vi "Read File+ [I16].vi"(6 "2D number of columns/1D count":i32 caption="2D-Spaltenanzahl/1D-Anzahl", 7 "2D number of rows":i32 caption="2D-Zeilenanzahl", 8 "error in (no error)":errorcluster caption="Fehler (Eingang, kein Fehler)", 9 "pos offset (bytes:0)":i32 caption="Pos.-Offset (Bytes:0)", 10 "pos mode (rel. to current:2)":enum16{"start", "end", "current"}(ring)=enum."current" caption="Pos.-Modus (relativ zur aktuellen Pos.:2)", 11 "refnum":refnum<file> caption="RefNum") -> (0 "error out":errorcluster caption="Fehler (Ausgang)", 1 "mark after read (bytes)":i32 caption="Dateimarke nach Lesevorgang (Byte)", 2 "1D data":i16[](array[numeric]) caption="1D Daten", 3 "2D data":i16[][](array[numeric]) caption="2D Daten", 4 "EOF?":bool caption="Dateiende?", 5 "dup refnum":refnum<file> caption="RefNum (Kopie)")   [LabVIEW 2009]
doc: "Liest ein 2D- oder 1D-Array von vorzeichenbehafteten Word-Integerzahlen (I16) an der angegebenen Position einer Byte-Stream-Datei aus; der voreingestellte Ort ist die aktuelle Markierung. Das VI überprüft eingehende und interne Fehler und liest nicht, wenn ein Eingangsfehler auftritt.\n\n'RefNum' ist die Referenz zur geöffneten Datei.\n\n'Pos.-Modus' legt fest, an welcher Stelle, relativ zu 'Pos.-Offset', zu schreiben begonnen wird:\n\n 0: am Anfang der Datei plus Pos.-Offest.\n\n 1: am Ende der Datei plus Pos.-Offest. \n\n 2: An der aktuellen Markierung plus Pos.-Offset. Dies ist die Standardeinstellung\n\nPos.-Offset legt in Byte fest, wie weit entfernt von Pos.-Modus begonnen wird. Die Voreinstellung ist 0. Byte-Einheiten sind flexibler als Integer(2 Byte)-Einheiten, Wenn eine Datei zum Beispiel einen Kopf, geschrieben mit Datei Schreiben+ (String) enthält, gefolgt von Array mit Zahlen aus Datei Schreiben+ [I16].\n\n2D-Zeilenanzahl ist die Anzahl der zu erzeugenden Zeilen, wenn Daten in ein 2D-Array eingelesen werden. Ist der Wert 0 (Standard), kommen die Daten im 1D-Array zurück.\n\n2D-Spaltenanzahl/1D-Werteanzahl ist die Anzahl der zu erstellenden Spalten, wenn die Daten in ein 2D-Array eingelesen werden, sofern die 2D-Zeilenanzahl größer 0 ist, oder es handelt sich um die Anzahl der in ein 1D-Array einzulesenden vorzeichenbehafteten Word-Integerzahlen.\n\nFehlereingang ist ein Cluster mit 3 Elementen (Fehler?, Code, und Quelle), das den bisherigen Fehlerstatus beschreibt, wenn bei vorher ausgeführten VIs ein Fehler aufgetreten ist. Trat kein Fehler auf, wird das VI normal ausgefürt; Trat ein Fehler auf, wird die Fehlermeldung weitergegeben. Fehler? ist TRUE wenn ein Fehler aufgetreten ist; die Voreinstellung ist FALSE. Code ist der Fehlercode; die Voreinstellung ist 0. Quelle ist in den meisten Fällen der Name des VIs oder der Funktion in der der Fehler aufgetreten ist; die Voreinstellung ist ein leerer String.\n\nRefNum (Kopie) ist ein weitergeleiteter Parameter, der den gleichen Wert wie RefNum hat.\n\n2D-Array enthält die aus der Datei gelesenen vorzeichenbehafteten Word-Integerzahlen, wenn die 2D-Zeilenanzahl gleich 0 ist; Andernfalls ist der Ausgang leer.\n\n1D-Array enthält die aus der Datei gelesenen vorzeichenbehafteten Word-Integerzahlen, wenn die 2D-Zeilenanzahl gleich 0 ist; Andernfalls ist der Ausgang leer.\n\nDateimarke nach Lesevorgang ist die Position der Dateimarke nach dem Lesen. Sie zeigt auf das Byte in der Datei, das auf das zuletzt gelesene Byte folgt.\n\nEOF? ist TRUE falls Sie versuchen nach dem Ende der Datei (EOF) zu lesen.\n\nFehlerausgang ist ein Cluster mit 3 Elementen (Fehler?, Code, und Quelle), das bei der Ausführung des VIs aufgetretene Fehler beschreibt. Wenn kein Eingangsfehler auftrat, wird das VI normal ausgeführt und der Fehlerausgang enthält den Fehlerstatus dieses VIs; wenn ein Eingangsfehler auftrat wird diesen an den Fehlerausgang weitergegeben."
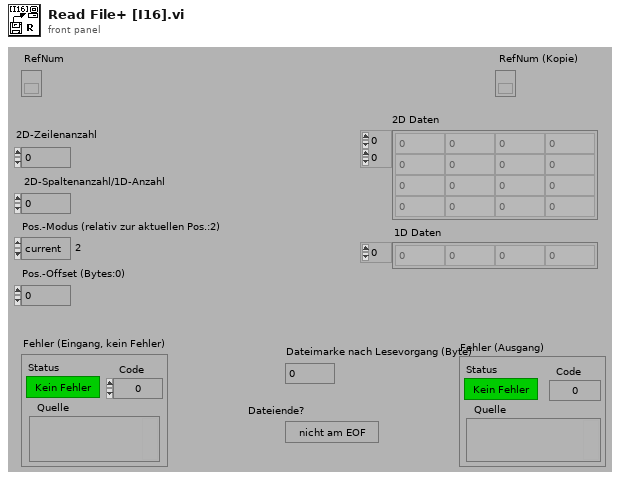
[diagram p1: front panel]
types:
  T1 = cluster{"2D number of rows":i32, "2D number of columns/1D count":i32}
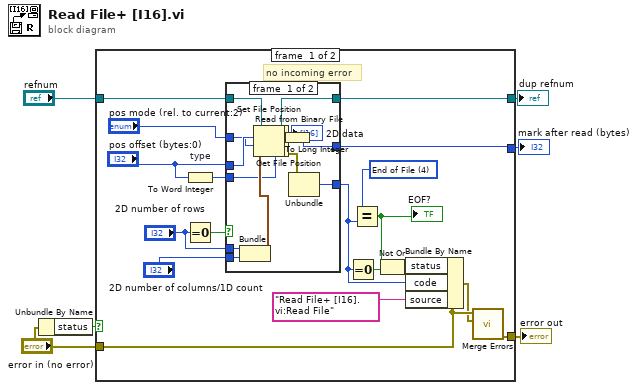
[diagram p0: block diagram]
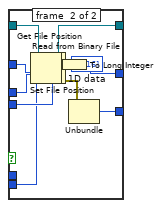
[diagram p2: hidden frame]
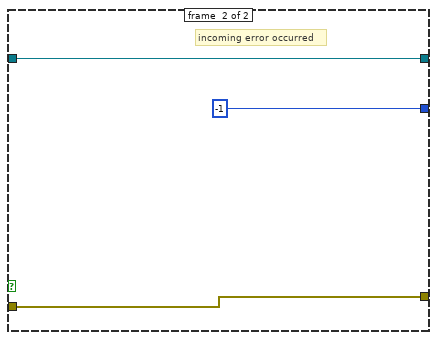
[diagram p3: hidden frame]
diagram:
  n1 = Unbundle By Name("error in (no error)") -> ("status"=w6:bool)
  n2 = case shown="False" w6 {
    tunnel: [w9 w58] -> w5
    tunnel: [w17 -1] -> w4
    tunnel: [w22 w57] -> w3
    tunnel: "refnum" -> [w21 w57]
    tunnel: "error in (no error)" -> [w8 w58]
    frame #0 {
      w11 = 4 items=["No Error", "Manager Argument Error", "Memory Full", "Out of Zone", "End of File", "File Already Open", "Generic File IO Error", "File Not Found", "File Permission Error", "Disk Full", "Duplicate Path", "Too Many Files Open", "Not Enabled", "Resource File Not Found", "Cannot Add Resource", "Resource Not Found", "Image Not Found", "Image Memory Error", "Pen Does Not Exist", "Config Bad Type", "Config Token Not Found", "Config Parse Error", "Config Memory Error", "Bad External Code Format", "Bad External Code Offset", "External Code Not Present", "Null Window", "Destroy Window Mixup", "Null Menu", "Print Aborted", "Bad Print Record", "Print Driver Error", "Windows Error During Print", "Memory Error During Print", "Print Dialog Error", "Generic Print Error", "Invalid Device Refnum", "Device Not Found", "Device Parameter Error", "Device Unit Error", "Can't Open Device", "Device Call Aborted", "Generic Error", "Cancelled By User", "Object ID Too Low", "Object ID Too High", "Object Not In Heap", "Unknown Heap", "Bad DefProc ID", "DefProc Not In Table", "Message Out Of Range", "Null Method", "Unknown Message", "Manager Call Not Supported"]
      # "no incoming error"
      n3 = To Word Integer "type"(number="pos offset (bytes:0)") -> (16bit integer=w24:i16)
      n4 = Equal To 0?(x="2D number of rows") -> (x = 0?=w23:bool)
      n5 = case shown="True" w23 {
        tunnel: [w32 w49] -> w13
        tunnel: [w36 w56] -> w17
        tunnel: w24 -> [w40 w55]
        tunnel: "2D number of columns/1D count" -> [w39 w50]
        tunnel: "2D number of rows" -> [w38 _]
        tunnel: [w35 w52] -> w22
        tunnel: w21 -> [w34 w53]
        tunnel: "pos mode (rel. to current:2)" -> [w30 w47]
        tunnel: "pos offset (bytes:0)" -> [w33 w51]
        frame #0 {
          n6 = Bundle("2D number of rows"=w38, "2D number of columns/1D count"=w39) -> (w41:T1)  [unwired: 1 in]
          n7 = Set File Position(offset (in bytes) (0)=w33, refnum=w34, from (0:start)=w30) -> (refnum out=w29:refnum<file>, error out=w28:errorcluster)  [unwired: 1 in]
          n8 = Read from Binary File(5:w40, 8:w28, 10:w41, 11:w29) -> (0:w26:errorcluster, 2:→"2D data":i16[][], 3:w27:refnum<file>)  [unwired: 2 in, 1 out]
          n9 = Get File Position(4:w26, 7:w27) -> (0:w31:errorcluster, 2:w25:i64, 3:w35:refnum<file>)
          n10 = To Long Integer(number=w25) -> (32bit integer=w36:i32)
          n11 = Unbundle(w31) -> ("code"=w32:i32)  [unwired: 2 out]
        }
        frame #1 {
          n12 = Set File Position(offset (in bytes) (0)=w51, refnum=w53, from (0:start)=w47) -> (refnum out=w46:refnum<file>, error out=w45:errorcluster)  [unwired: 1 in]
          n13 = Read from Binary File(5:w55, 8:w45, 10:w50, 11:w46) -> (0:w43:errorcluster, 2:→"1D data":i16[], 3:w44:refnum<file>)  [unwired: 2 in, 1 out]
          n14 = Get File Position(4:w43, 7:w44) -> (0:w48:errorcluster, 2:w42:i64, 3:w52:refnum<file>)
          n15 = To Long Integer(number=w42) -> (32bit integer=w56:i32)
          n16 = Unbundle(w48) -> ("code"=w49:i32)  [unwired: 2 out]
        }
      }
      n17 = Equal To 0?(x=w13) -> (x = 0?=w15:bool)
      n18 = Equal?(x=w11, y=w13) -> (x = y?=w14:bool)
      "EOF?" <- w14
      n19 = Not Or(1:w15, 2:w14) -> (0:w10:bool)
      n20 = Bundle By Name(cluster=w8, "status"=w10, "code"=w13, "source"="Read File+ [I16].vi:Read File") -> (w7:errorcluster)
      n21 = call <vilib>:"Merge Errors.vi"("error in 2 (no error)"=w7, "error in 1 (no error)"=w8) -> ("error out"=w9:errorcluster)  [unwired: 5 in]
    }
    frame #1 {
      # "incoming error occurred"
    }
  }
  "error out" <- w5
  "mark after read (bytes)" <- w4
  "dup refnum" <- w3
